vi "Test Amplitude Class.vi"(8 "error in (no error)":errorcluster, 11 "TestCase in":refnum<class "Test FGEN.lvclass">) -> (0 "error out":errorcluster, 3 "TestCase out":refnum<class "Test FGEN.lvclass">)   [LabVIEW 2020, in "Test FGEN.lvclass"]
uses:
  Test FGEN.lvclass
  Libraries/FGen/Generador/Generador.lvclass
  Libraries/FGen/GeneradorAmplificado/GeneradorAmplificado.lvclass
  C:/Users/ronad/IVAbraham2P/Libraries/FGen/Generador/Generador.lvclass
  <vilib>/measure/mascope.llb/Amplitude and Levels 1 chan.vi
  <vilib>/addons/_JKI Toolkits/VI Tester/TestCase.llb/TestCase.lvclass
  <vilib>/measure/NI_MAPro.lvlib
  C:/Program Files (x86)/National Instruments/LabVIEW 2020/vi.lib/addons/_JKI Toolkits/VI Tester/TestCase.llb/TestCase.lvclass
panel:
  out "Array":dbl[](array[numeric])
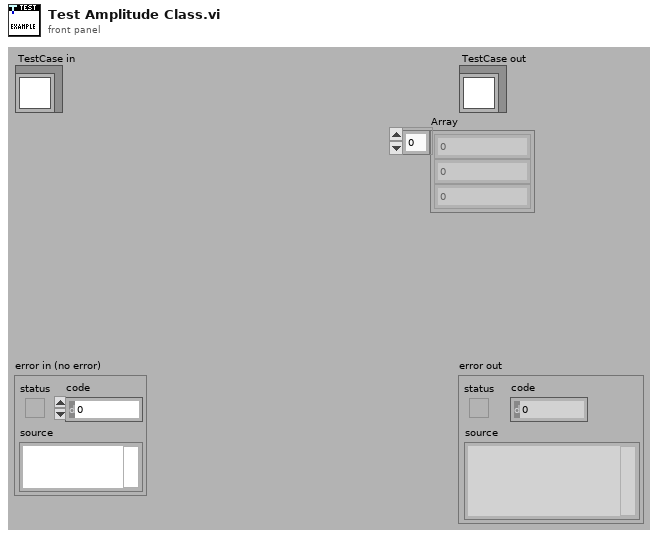
[diagram p1: front panel]
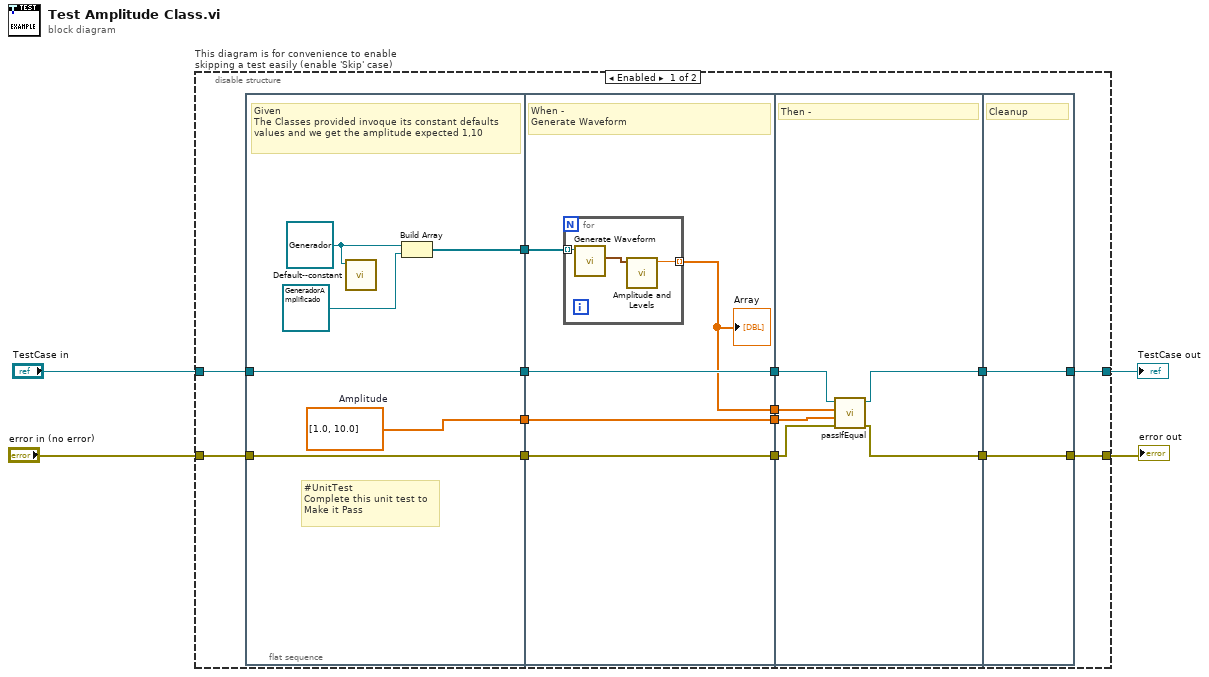
[diagram p0: block diagram]
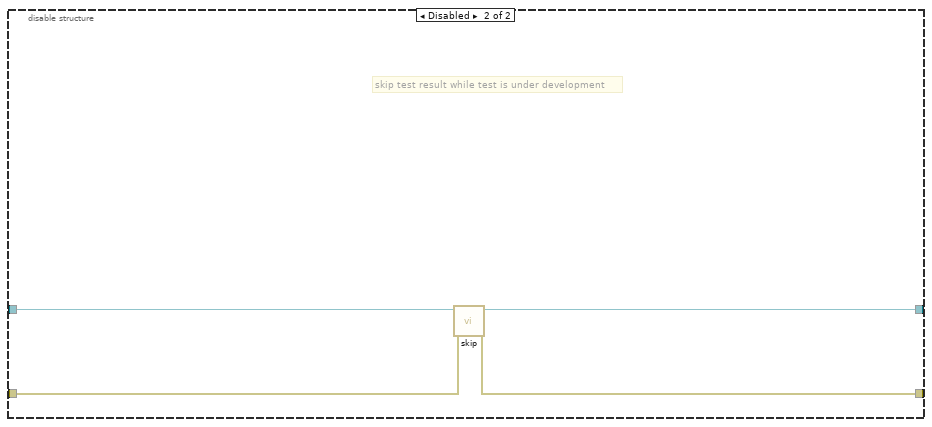
[diagram p2: hidden frame]
diagram:
  n1 = disable-structure "This diagram is for convenience to enable skipping a test easily (enable 'Skip' case)" shown="Enabled" {
    disable-tunnel: "TestCase in" -> [w14 w44]
    disable-tunnel: [w12 w42] -> w1
    disable-tunnel: [w13 w43] -> w3
    disable-tunnel: "error in (no error)" -> [w11 w41]
    frame Enabled {
      n2 = flat-sequence {
        tunnel: w14 -> [w24]
        tunnel: [w24] -> w18
        tunnel: w11 -> [w23]
        tunnel: [w23] -> w9
        tunnel: [w22] -> w7
        tunnel: [w21] -> w5
        tunnel: [w29] -> w17
        tunnel: w18 -> [w29]
        tunnel: [w28] -> w10
        tunnel: w9 -> [w28]
        tunnel: [w27] -> w8
        tunnel: w7 -> [w26]
        tunnel: [w26] -> w6
        tunnel: w5 -> [w25]
        tunnel: [w37] -> w16
        tunnel: [w36] -> w15
        tunnel: w17 -> [w38]
        tunnel: w10 -> [w35]
        tunnel: w8 -> [w34]
        tunnel: w6 -> [w33]
        tunnel: [w39] -> w13
        tunnel: [w40] -> w12
        tunnel: w16 -> [w40]
        tunnel: w15 -> [w39]
        frame #0 {
          w22 = dbl[] [1.0, 10.0]  # Amplitude
          w19 = refnum<class "Generador.lvclass"> refnum ("FGen.lvlib:Generator")
          # "#UnitTest\nComplete this unit test to\nMake it Pass"
          # "Given\nThe Classes provided invoque its constant defaults values and we get the amplitude expected 1,10"
          n3 = call-dynamic "Default--constant.vi"("Generator in"=w19) -> ()  [unwired: 9 in, 2 out]
          n4 = Build Array(w19, refnum<class "GeneradorAmplificado.lvclass"> refnum ("FGen.lvlib:GeneradorAmplificado.lvclass")) -> (w21:refnum<class "Generador.lvclass">[])
        }
        frame #1 {
          # "When -\nGenerate Waveform"
          n5 = for {
            tunnel: [w31] -> w27 mode=indexing
            tunnel: w25 -> [w30] mode=indexing
            n6 = call "Generate Waveform.vi"("Generator in"=w30) -> ("Waveform"=w32:waveform(dbl))  [unwired: 8 in, 2 out]
            n7 = call-poly <vilib>:"Amplitude and Levels.vi"("signal in"=w32) -> ("amplitude"=w31:dbl)  [unwired: 7 in, 3 out]
          }
          "Array" <- w27
        }
        frame #2 {
          # "Then -"
          n8 = call-dynamic "passIfEqual.vi"("error in (no error)"=w35, "y"=w33, "x"=w34, "TestCase in"=w38) -> ("error out"=w36:errorcluster, "TestCase out"=w37:refnum<class "Test FGEN.lvclass">)  [unwired: 6 in]
        }
        frame #3 {
          # "Cleanup"
        }
      }
    }
    frame Disabled {
      # "skip test result while test is under development"
      n9 = call <vilib>:"skip.vi"("error in (no error)"=w41, "TestCase in"=w44) -> ("error out"=w43:errorcluster, "TestCase out"=w42:refnum<class "Test FGEN.lvclass">)  [unwired: 8 in]
    }
  }
  "error out" <- w3
  "TestCase out" <- w1
